vi "ProcessAudioFile.vi"(7 "Qbus in":refnum<class "Qbus.lvclass">, 8 "error in (no error)":errorcluster, 10 "data":T1, 11 "config in":T2={"DataSet Type"=enum."Waveform", "ChanNameMap"=variant, "Common"={"State"=enum."On", "Waveform Channel"="", "DataGroup"="", "Number of Samples"=0, "Waveform Length (sec)"=0.0, "Timeout"=0.0, "History"=variant, "LastRequest"=timestamp(0 s since 1904-01-01), "BufferSize"=0, "OpState"=variant, "IRoutingSource"={"CorrelationId"="", "ReplyTo"=""}}}) -> (0 "error out":errorcluster, 3 "config out":T2={"DataSet Type"=enum."Waveform", "ChanNameMap"=variant, "Common"={"State"=enum."On", "Waveform Channel"="", "DataGroup"="", "Number of Samples"=0, "Waveform Length (sec)"=0.0, "Timeout"=0.0, "History"=variant, "LastRequest"=timestamp(0 s since 1904-01-01), "BufferSize"=0, "OpState"=variant, "IRoutingSource"={"CorrelationId"="", "ReplyTo"=""}}})   [LabVIEW 2017, in "EmsaTestPanel.lvlib"]
uses:
  <vilib>/addons/InsightCM/Devices/Shared/Emsa/EmsaTestPanel/EmsaTestPanel.lvlib
  <vilib>/addons/InsightCM/Devices/Shared/Emsa/EmsaTestPanel/controls/Configuration.ctl
  <vilib>/addons/InsightCM/Devices/Shared/Emsa/EmsaTestPanel/controls/DataSetType.ctl
  <vilib>/addons/InsightCM/Devices/Shared/Common/TestPanel/controls/Configuration.ctl
  <vilib>/addons/InsightCM/Devices/Shared/Common/TestPanel/controls/State.ctl
  <vilib>/addons/InsightCM/MessageBus/Base/controls/IRoutingSource.ctl
  <vilib>/addons/Qbus/Qbus.lvclass
  <vilib>/addons/InsightCM/Devices/Shared/Emsa/EmsaAudio/controls/AudioFileCompleteBroadcast.ctl
  <vilib>/addons/InsightCM/MessageBus/MessageLibrary/Device/controls/DeviceTestPanelGetDataSetForChannelResponseBody.ctl
  <vilib>/addons/InsightCM/MessageBus/Base/controls/DataSetByteData.ctl
  <vilib>/addons/InsightCM/MessageBus/Base/controls/KeyValuePair.ctl
  <vilib>/addons/InsightCM/Devices/Shared/Common/ServerComm/ServerComm.lvlib
  <vilib>/addons/InsightCM/Devices/Shared/Common/TestPanel/TestPanel.lvlib
  <vilib>/addons/InsightCM/Devices/Shared/Emsa/EmsaAudio/EmsaAudio.lvlib
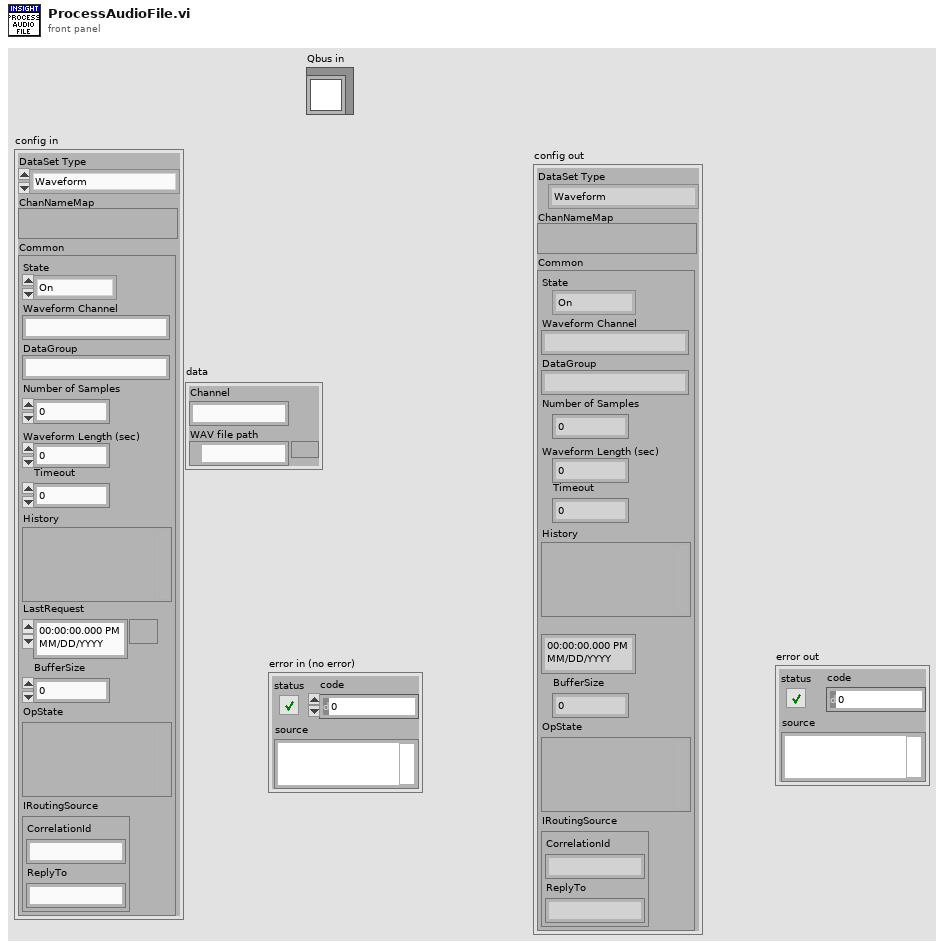
[diagram p1: front panel]
types:
  T1 = typedef "EmsaAudio.lvlib/AudioFileCompleteBroadcast.ctl" = cluster{"Channel":string, "WAV file path":path}
  T2 = typedef "EmsaTestPanel.lvlib/Configuration.ctl" = cluster{"DataSet Type":T3, "ChanNameMap":variant, "Common":T4}
  T3 = typedef "EmsaTestPanel.lvlib/DataSetType.ctl" = enum16{"Waveform", "Sweep", "WAV"}
  T4 = typedef "TestPanel.lvlib/Configuration.ctl" = cluster{"State":T5, "Waveform Channel":string, "DataGroup":string, "Number of Samples":i32, "Waveform Length (sec)":dbl, "Timeout":dbl, "History":variant, "LastRequest":timestamp, "BufferSize":i32, "OpState":variant, "IRoutingSource":T6}
  T5 = typedef "TestPanel.lvlib/State.ctl" = enum16{"Off", "On", "PendingValues", "PendingDataSet"}
  T6 = typedef "IRoutingSource.ctl" = cluster{"CorrelationId":string, "ReplyTo":string}
  T7 = typedef "DeviceTestPanelGetDataSetForChannelResponseBody.ctl" = cluster{"DataSet":T8}
  T8 = typedef "DataSetByteData.ctl" = cluster{"Id":string, "DataEventId":string, "AssetNodeId":string, "Type":string, "T0":i64, "Props":T9[], "DataBase64":string}
  T9 = typedef "KeyValuePair.ctl" = cluster{"Key":string, "Value":string}
  T10 = typedef "Message.ctl" = cluster{"Header":T11, "Body":u8[]}
  T11 = typedef "MessageHeader.ctl" = cluster{"MessageName":string, "Timestamp":i64, "CorrelationId":string, "ContentType":string, "RoutingKey":string, "Properties":T9[]}
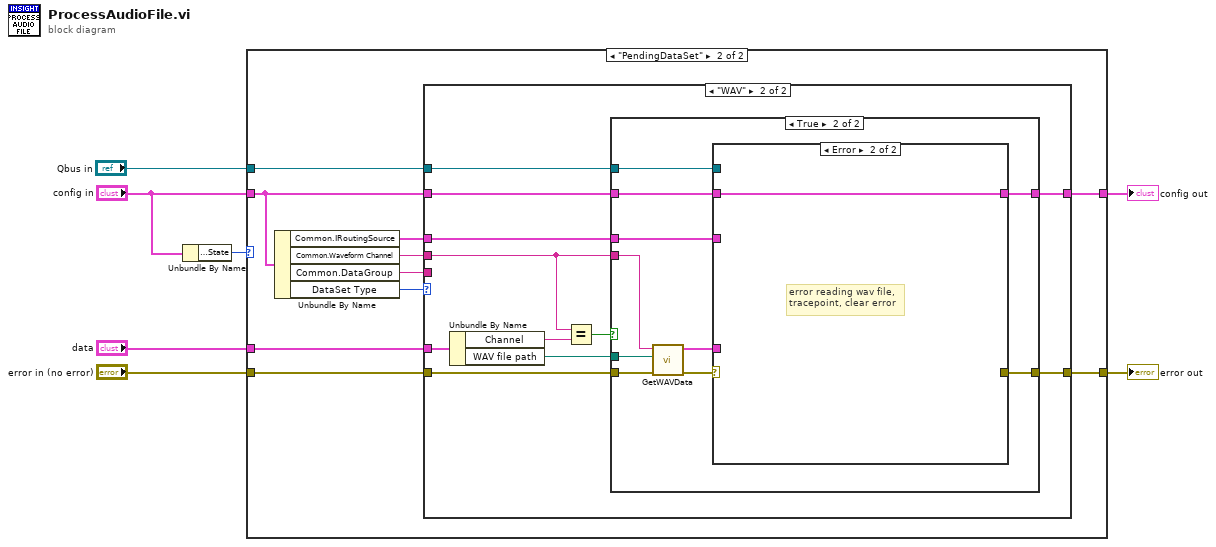
[diagram p0: block diagram]
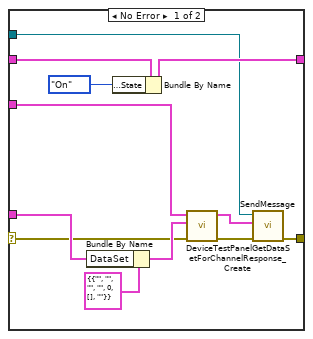
[diagram p5: hidden frame]
diagram:
  n1 = Unbundle By Name("config in") -> ("Common.State"=w7:T5)
  n2 = case shown="\"PendingDataSet\"" w7 {
    tunnel: "error in (no error)" -> [w8 w19]
    tunnel: [w8 w14] -> w3
    tunnel: "config in" -> [w9 w17]
    tunnel: [w9 w16] -> w4
    tunnel: "Qbus in" -> [_ w15]
    tunnel: "data" -> [_ w10]
    frame Default {
    }
    frame "PendingDataSet" {
      n3 = Unbundle By Name(w17) -> ("Common.IRoutingSource"=w13:T6, "Common.Waveform Channel"=w18:string, "Common.DataGroup"=w12:string, "DataSet Type"=w11:T3)
      n4 = case shown="\"WAV\"" w11 {
        tunnel: w19 -> [w20 w32]
        tunnel: w18 -> [_ w25]
        tunnel: w17 -> [w21 w31]
        tunnel: [w21 w30] -> w16
        tunnel: w15 -> [_ w29]
        tunnel: [w20 w28] -> w14
        tunnel: w13 -> [_ w27]
        tunnel: w12 -> [_ _]
        tunnel: w10 -> [_ w26]
        frame Default {
        }
        frame "WAV" {
          n5 = Unbundle By Name(w26) -> ("Channel"=w24:string, "WAV file path"=w22:path)
          n6 = Equal?(x=w25, y=w24) -> (x = y?=w23:bool)
          n7 = case shown="True" w23 {
            tunnel: w32 -> [w34 w38]
            tunnel: w25 -> [_ w39]
            tunnel: w31 -> [w33 w44]
            tunnel: [w33 w43] -> w30
            tunnel: w29 -> [_ w42]
            tunnel: [w34 w41] -> w28
            tunnel: w27 -> [_ w40]
            tunnel: w22 -> [_ w36]
            frame False {
            }
            frame True {
              n8 = call <vilib>:"GetWAVData.vi"("error in (no error)"=w38, "WAV file path"=w36, "Channel"=w39) -> ("error out"=w35:errorcluster, "DataSet"=w37:T8)  [unwired: 7 in]
              n9 = case shown="Error" w35 {
                selector: w35 -> [w45 _]
                tunnel: w44 -> [w56 w57]
                tunnel: [w55 w57] -> w43
                tunnel: w42 -> [w54 _]
                tunnel: [w51 _] -> w41
                tunnel: w40 -> [w49 _]
                tunnel: w37 -> [w46 _]
                frame No Error {
                  n10 = Bundle By Name(cluster=T7 {"DataSet"={"Id"="", "DataEventId"="", "AssetNodeId"="", "Type"="", "T0"=0, "Props"=[], "DataBase64"=""}} ("DeviceTestPanelGetWaveformChannelResponse"), "DataSet"=w46) -> (w50:T7)
                  n11 = Bundle By Name(cluster=w56, "Common.State"=State."On" ("Test Panel State")) -> (w55:T2)
                  n12 = call <vilib>:"DeviceTestPanelGetDataSetForChannelResponse_Create.vi"("error in (no error)"=w45, "DeviceTestPanelGetDataSetForChannelResponse"=w50, "IRoutingSource"=w49) -> ("error out"=w52:errorcluster, "Message"=w48:T10)  [unwired: 7 in]
                  n13 = call <vilib>:"SendMessage.vi"("error in (no error)"=w52, "message"=w48, "Qbus in"=w54) -> ("error out"=w51:errorcluster)  [unwired: 7 in, 1 out]
                }
                frame Error {
                  # "error reading wav file,\ntracepoint, clear error"
                }
              }
            }
          }
        }
      }
    }
  }
  "error out" <- w3
  "config out" <- w4
